vi "Read convertPtoQ.vi"(8 "error in (no error)":errorcluster, 11 "P in":refnum<class "P.lvclass">) -> (0 "error out":errorcluster, 2 "convertPtoQ":bool, 3 "P out":refnum<class "P.lvclass">)   [LabVIEW 2015, in "P.lvclass"]
uses:
  P.lvclass
  P.lvclass/P.ctl
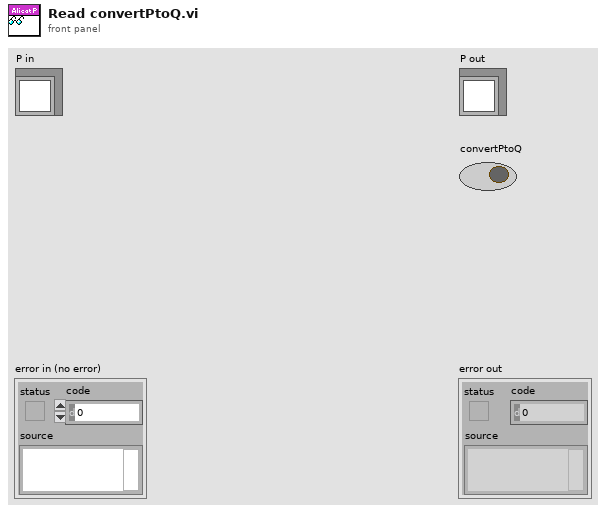
[diagram p1: front panel]
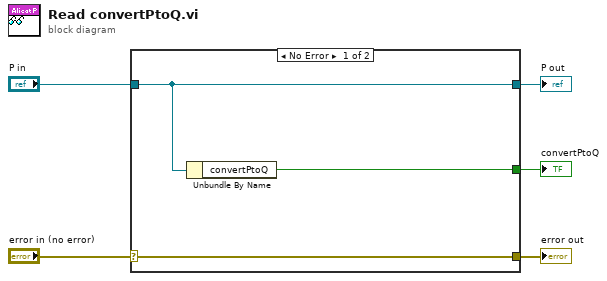
[diagram p0: block diagram]
diagram:
  n1 = case shown="No Error" "error in (no error)" {
    selector: "error in (no error)" -> [w8 w9]
    tunnel: [w8 w9] -> w4
    tunnel: [w7 w10] -> w2
    tunnel: "P in" -> [w7 w10]
    tunnel: [w6 _] -> w1
    frame No Error {
      n2 = Unbundle By Name(w7) -> ("convertPtoQ"=w6:bool)
    }
    frame Error {
    }
  }
  "error out" <- w4
  "P out" <- w2
  "convertPtoQ" <- w1
